vi "GetFrame.vi"(8 "error in (no error)":errorcluster, 10 "Image In":T1, 11 "Hamamatsu_Camera in":refnum<class "Hamamatsu_Camera.lvclass">) -> (0 "error out":errorcluster, 3 "Hamamatsu_Camera out":refnum<class "Hamamatsu_Camera.lvclass">)   [LabVIEW 2023, in "Hamamatsu_Camera.lvlib" / "Hamamatsu_Camera.lvclass"]
uses:
  Hamamatsu_Camera.lvclass
  <vilib>/vision/Image Controls.llb/IMAQ Image.ctl
  Hamamatsu_Camera.lvclass/Hamamatsu_Camera.ctl
  Interfaces/AbstractInstrumentClasses/Cameras_LV/CameraComm Messages/Frame Ready Msg/Frame Ready Msg.lvclass/Frame Ready Msg.ctl
  <vilib>/ActorFramework/Message Enqueuer/Message Enqueuer.lvclass/Message Enqueuer.ctl
  <vilib>/ActorFramework/Message Enqueuer/Enqueue.vi
  Interfaces/AbstractInstrumentClasses/Cameras_LV/CameraComm Messages/Frame Ready Msg/Frame Ready Msg.lvclass
  C:/Program Files/National Instruments/LabVIEW 2023/vi.lib/ActorFramework/Message/Message.lvclass
  <vilib>/ActorFramework/Message Priority Queue/Priority Enqueue.vi
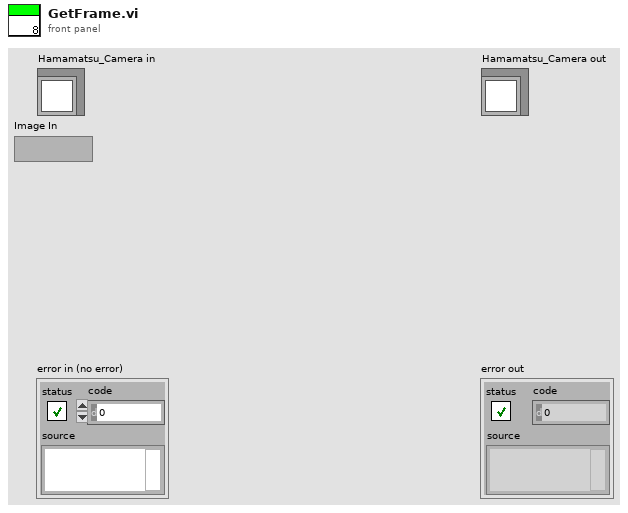
[diagram p1: front panel]
types:
  T1 = typedef "IMAQ Image.ctl" = refnum<image>
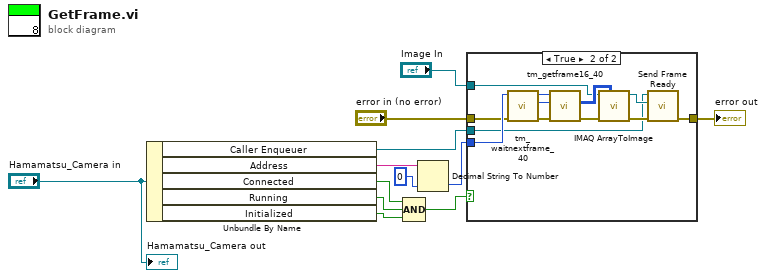
[diagram p0: block diagram]
diagram:
  n1 = Unbundle By Name("Hamamatsu_Camera in") -> ("Caller Enqueuer"=w1:refnum<class "Message Enqueuer.lvclass">, "Address"=w11:string, "Connected"=w5:bool, "Running"=w4:bool, "Initialized"=w3:bool)
  n2 = Compound Arithmetic op=AND(w5, w4, w3) -> (w2:bool)
  n3 = Decimal String To Number(string=w11, default (0L)=u32 0 ("default (0 I32)")) -> (number=w8:u32)  [unwired: 1 in, 1 out]
  n4 = case shown="True" w2 {
    tunnel: "Image In" -> [_ w20]
    tunnel: w8 -> [_ w19]
    tunnel: "error in (no error)" -> [w13 w18]
    tunnel: [w13 w15] -> w6
    tunnel: w1 -> [_ w14]
    frame False {
    }
    frame True {
      n5 = call "tm_waitnextframe_40.vi"("error in (no error)"=w18, "Handle in"=w19) -> ("error out"=w25:errorcluster, "Frame Index"=w23:i32, "Handle out"=w24:u32)  [unwired: 6 in, 1 out]
      n6 = call "tm_getframe16_40.vi"("error in (no error)"=w25, "Frame Index"=w23, "Handle in"=w24) -> ("error out"=w21:errorcluster, "Data"=w22:u16[][])  [unwired: 5 in, 2 out]
      n7 = call "IMAQ ArrayToImage"("Image Pixels (U16)"=w22, "error in (no error)"=w21, "Image"=w20) -> ("error out"=w16:errorcluster, "Image Out"=w17:T1)  [unwired: 7 in]
      n8 = call "Send Frame Ready.vi"("error in (no error)"=w16, "Image In"=w17, "Message Enqueuer"=w14) -> ("error out"=w15:errorcluster)  [unwired: 7 in, 1 out]
    }
  }
  "error out" <- w6
  "Hamamatsu_Camera out" <- "Hamamatsu_Camera in"
